vi "Configure IP Address.vi"(8 "error in (no error)":errorcluster, 10 "IP Address (100.100.100.100)":string="100.100.100.100", 11 "VISA resource name":refnum<visa-resource-name>) -> (0 "error out":errorcluster, 3 "VISA resource name out":refnum<visa-resource-name>)   [LabVIEW 2014, in "Associated Research SC6540.lvlib"]
doc: "Sets the IP Address of the instrument"
uses:
  <instrlib>/Associated Research SC6540/Associated Research SC6540.lvlib
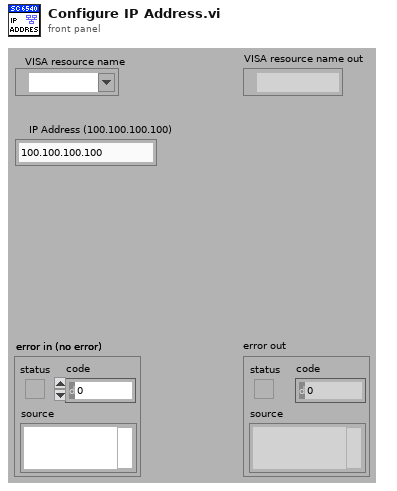
[diagram p1: front panel]
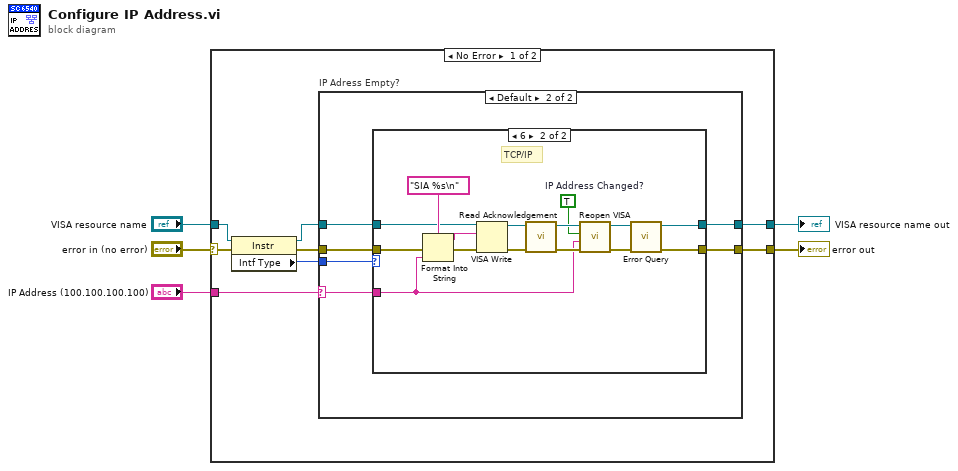
[diagram p0: block diagram]
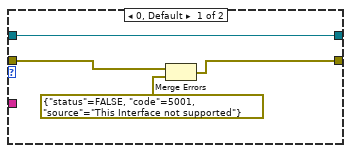
[diagram p3: hidden frame]
diagram:
  n1 = case shown="No Error" "error in (no error)" {
    selector: "error in (no error)" -> [w11 w42]
    tunnel: "VISA resource name" -> [w9 w41]
    tunnel: [w13 w41] -> w5
    tunnel: [w12 w42] -> w4
    tunnel: "IP Address (100.100.100.100)" -> [w6 _]
    frame No Error {
      n2 = property class="Instr"(reference=w9, error in=w11) -> (reference out=w8:refnum<visa-resource-name>, error out=w10:errorcluster, "Intf Type"=w7:u16)
      n3 = case "IP Adress Empty?" shown="Default" w6 {
        selector: w6 -> [_ w16]
        tunnel: [w14 w21] -> w13
        tunnel: [w15 w20] -> w12
        tunnel: w10 -> [w15 w19]
        tunnel: w8 -> [w14 w18]
        tunnel: w7 -> [_ w17]
        frame "" {
        }
        frame Default {
          n4 = case shown="6" w17 {
            tunnel: [w25 w40] -> w21
            tunnel: [w23 w38] -> w20
            tunnel: w19 -> [w22 w32]
            tunnel: w18 -> [w25 w31]
            tunnel: w16 -> [_ w26]
            frame 0, Default {
              n5 = Merge Errors(w22, errorcluster {"status"=FALSE, "code"=5001, "source"="This Interface not supported"} ("error in 2 (no error)")) -> (w23:errorcluster)
            }
            frame 6 {
              w27 = TRUE  # IP Address Changed?
              # "TCP/IP"
              n6 = Format Into String(format string="SIA %s\n" ("Command to Send"), error in=w32, w26) -> (resulting string=w37:string, error out=w36:errorcluster)  [unwired: 1 in]
              n7 = VISA Write(VISA resource name=w31, write buffer=w37, error in (no error)=w36) -> (VISA resource name out=w33:refnum<visa-resource-name>, error out=w39:errorcluster)  [unwired: 1 out]
              n8 = call <instrlib>:"Read Acknowledgement.vi"("error in (no error)"=w39, "VISA resource name"=w33) -> ("error out"=w34:errorcluster, "VISA resource name out"=w29:refnum<visa-resource-name>)  [unwired: 8 in]
              n9 = call <instrlib>:"Reopen VISA.vi"("error in (no error)"=w34, "IP Address (000.000.000.000)"=w26, "Enable IP Address Changed (F: Disable)"=w27, "VISA resource name"=w29) -> ("error out"=w30:errorcluster, "VISA resource name out"=w28:refnum<visa-resource-name>)  [unwired: 6 in]
              n10 = call <instrlib>:"Error Query.vi"("error in (no error)"=w30, "VISA resource name"=w28) -> ("error out"=w38:errorcluster, "VISA resource name out"=w40:refnum<visa-resource-name>)  [unwired: 6 in, 2 out]
            }
          }
        }
      }
    }
    frame Error {
    }
  }
  "error out" <- w4
  "VISA resource name out" <- w5
